vi "DO_所有参数读取.vi"(8 "error in (no error)":errorcluster caption="错误输入（无错误）", 11 "MB session in":refnum<class "MB_Master.lvclass">) -> (0 "error out":errorcluster caption="错误输出", 2 "输出值":T1 {"电极型号标志" items=["NULL", "pH", "Cond", "DO", "Turb"]; "电极状态标志" items=["OK"]}, 3 "MB session out":refnum<class "MB_Master.lvclass">)   [LabVIEW 2016, in "斯坦道多参数.lvlib"]
uses:
  <vilib>/Plasmionique/MB Master/MB_Master/MB_Master.lvclass
  <vilib>/Plasmionique/MB Master/MB Master.lvlib
  <vilib>/ptbypt/NI_PtbyPt.lvlib
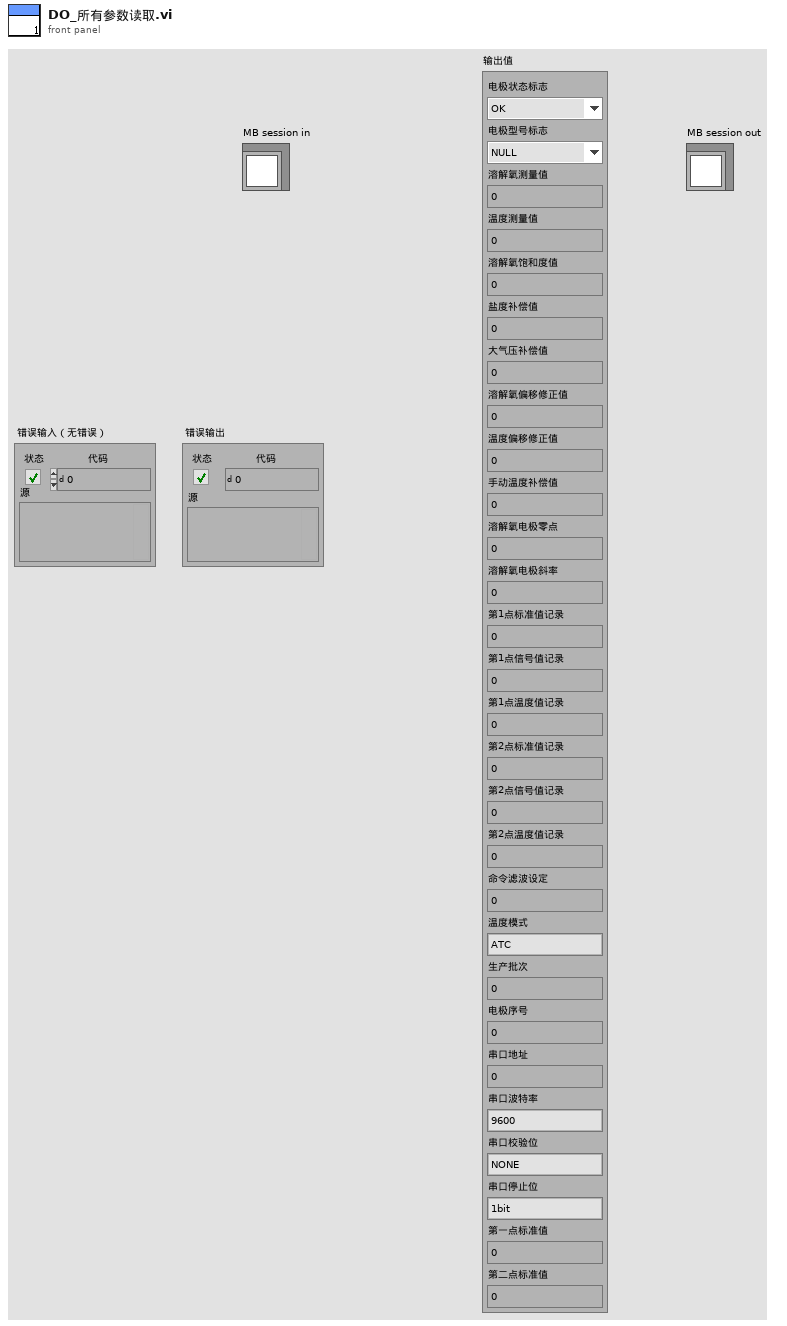
[diagram p1: front panel]
types:
  T1 = cluster{"电极状态标志":u16, "电极型号标志":u16, "溶解氧测量值":sgl, "温度测量值":sgl, "溶解氧饱和度值":sgl, "盐度补偿值":sgl, "大气压补偿值":sgl, "溶解氧偏移修正值":sgl, "温度偏移修正值":sgl, "手动温度补偿值":sgl, "溶解氧电极零点":sgl, "溶解氧电极斜率":sgl, "第1点标准值记录":sgl, "第1点信号值记录":sgl, "第1点温度值记录":sgl, "第2点标准值记录":sgl, "第2点信号值记录":sgl, "第2点温度值记录":sgl, "命令滤波设定":u16, "温度模式":enum16{"ATC", "MTC"}, "生产批次":u16, "电极序号":u16, "串口地址":u16, "串口波特率":enum16{"9600", "19200", "115200"}, "串口校验位":enum16{"NONE", "ODD", "EVEN"}, "串口停止位":enum16{"1bit", "2bit"}, "第一点标准值":sgl, "第二点标准值":sgl}
  T2 = cluster{u16, u16, "Filtered x":dbl, "数值":sgl, "数值":sgl, "数值":sgl, "数值":sgl, "数值":sgl, "数值":sgl, "数值":sgl, "数值":sgl, "数值":sgl, "数值":sgl, "数值":sgl, "数值":sgl, "数值":sgl, "数值":sgl, "数值":sgl, u16, u16, u16, u16, u16, u16, u16, u16, "数值":sgl, "数值":sgl}
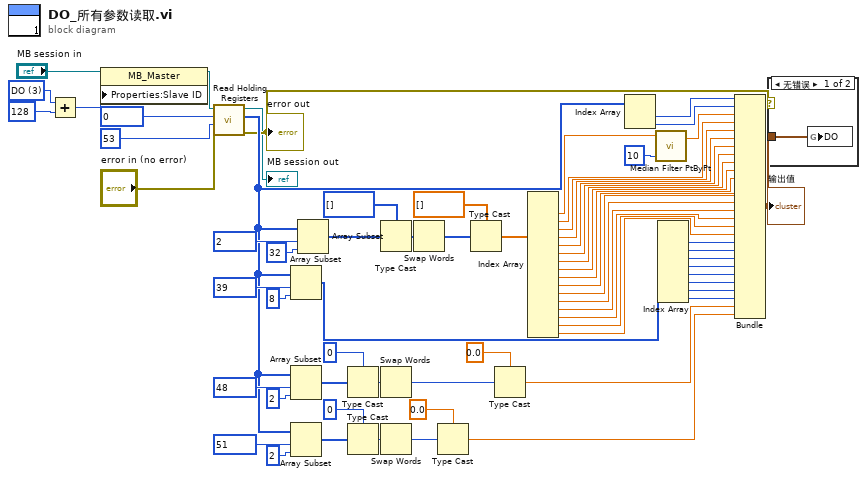
[diagram p0: block diagram]
diagram:
  w67 = u16 3 items=["NULL", "pH", "Cond", "DO", "Turb"] ("数值")
  n1 = Add(x=w67, y=u16 128) -> (x+y=w66:u16)
  n2 = property class="MB_Master"(reference="MB session in", "Properties:Slave ID"=w66) -> (reference out=w12:refnum<class "MB_Master.lvclass">)  [unwired: 1 in, 1 out]
  n3 = call <vilib>:"Read Holding Registers.vi"("error in (no error)"="error in (no error)", "quantity"=u16 53, "starting address"=u16 0, "MB session in"=w12) -> ("error out"=w7:errorcluster, "Registers"=w26:u16[], "MB session out"=→"MB session out":refnum<class "MB_Master.lvclass">)  [unwired: 5 in]
  "error out" <- w7
  n4 = Array Subset(array=w26, index=u16 39 ("starting address"), length=8 ("长度")) -> (w39:u16[])
  n5 = Array Subset(array=w26, index=u16 48 ("starting address"), length=2 ("长度")) -> (w21:u16[])
  n6 = Array Subset(array=w26, index=u16 51 ("starting address"), length=2 ("长度")) -> (w16:u16[])
  n7 = Array Subset(array=w26, index=u16 2 ("starting address"), length=32 ("长度")) -> (w55:u16[])
  n8 = Type Cast(type=u32 0 ("数值"), x=w21) -> (*(type *) &x=w24:u32)
  n9 = Type Cast(type=u32 0 ("数值"), x=w16) -> (*(type *) &x=w18:u32)
  n10 = Type Cast(type=u32[] [] ("数组 2"), x=w55) -> (*(type *) &x=w58:u32[])
  n11 = Swap Words(1:w24) -> (0:w25:u32)
  n12 = Swap Words(1:w18) -> (0:w17:u32)
  n13 = Swap Words(1:w58) -> (0:w59:u32[])
  n14 = Type Cast(type=sgl 0.0 ("数值"), x=w17) -> (*(type *) &x=w14:sgl)
  n15 = Type Cast(type=sgl[] [] ("数组 2"), x=w59) -> (*(type *) &x=w54:sgl[])
  n16 = Type Cast(type=sgl 0.0 ("数值"), x=w25) -> (*(type *) &x=w15:sgl)
  n17 = Index Array(array=w54) -> (element #1=w2:sgl, element #2=w8:sgl, element #3=w9:sgl, element #4=w10:sgl, element #5=w11:sgl, element #6=w53:sgl, element #7=w52:sgl, element #8=w51:sgl, element #9=w50:sgl, element #10=w49:sgl, element #11=w48:sgl, element #12=w47:sgl, element #13=w46:sgl, element #14=w45:sgl, element #15=w44:sgl, element #16=w43:sgl)  [unwired: 16 in]
  n18 = Index Array(array=w26) -> (element #1=w62:u16, element #2=w61:u16)  [unwired: 2 in]
  n19 = call <vilib>:"Median Filter PtByPt.vi"("rank"=10, "x"=w2) -> ("Filtered x"=w1:dbl)  [unwired: 2 in, 1 out]
  n20 = Index Array(array=w39) -> (element #1=w38:u16, element #2=w37:u16, element #3=w36:u16, element #4=w35:u16, element #5=w34:u16, element #6=w33:u16, element #7=w32:u16, element #8=w31:u16)  [unwired: 8 in]
  n21 = Bundle(w62, w61, "Filtered x"=w1, "数值"=w8, "数值"=w9, "数值"=w10, "数值"=w11, "数值"=w53, "数值"=w52, "数值"=w51, "数值"=w50, "数值"=w49, "数值"=w48, "数值"=w47, "数值"=w46, "数值"=w45, "数值"=w44, "数值"=w43, w38, w37, w36, w35, w34, w33, w32, w31, "数值"=w15, "数值"=w14) -> (w6:T2)  [unwired: 1 in]
  "输出值" <- w6
  n22 = case shown="无错误" w7 {
    tunnel: w6 -> [w68 _]
    frame No Error {
      n23 = global write "国弘过程全局变量.vi" "DO"(w68) -> ()
    }
    frame Error {
    }
  }
